vi "RDS Msg To String.vi"(8 "error in (no error)":errorcluster, 11 "String Message in":refnum<class "String Message.lvclass">) -> (0 "error out":errorcluster, 2 "String":string, 3 "String Message out":refnum<class "String Message.lvclass">)   [LabVIEW 2015, in "RDS Child Messages.lvlib" / "String Message.lvclass"]
uses:
  String Message.lvclass
  String Message.lvclass/String Message.ctl
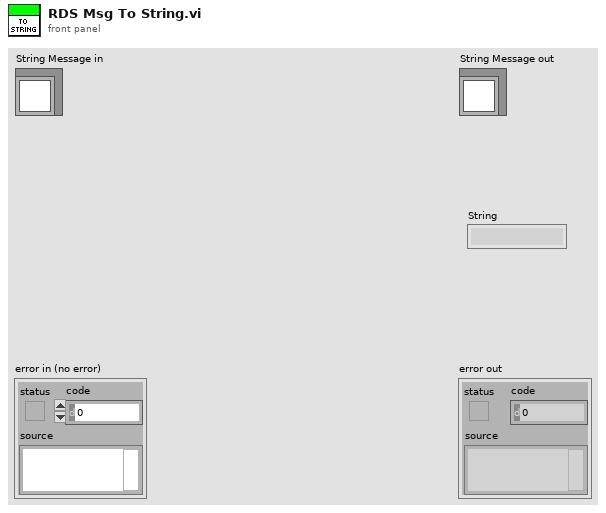
[diagram p1: front panel]
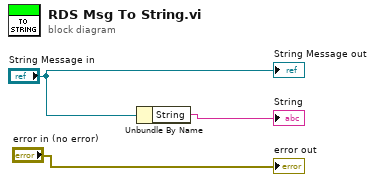
[diagram p0: block diagram]
diagram:
  n1 = Unbundle By Name("String Message in") -> ("String"=→"String":string)
  "error out" <- "error in (no error)"
  "String Message out" <- "String Message in"
